vi "ADD to DRIVE.vi"(11 "zero v":T2[](array[typedef])=[{"identifier"=2, "extended?"=FALSE, "type"=0, "payload"=[1, 0, 0, 0, 0, 0, 0]}, {"identifier"=2, "extended?"=FALSE, "type"=0, "payload"=[1]}] {"type" items=["CAN Data", "CAN Remote"]; "identifier" format="%.0x"}) -> (3 "Message Cluster":T1)   [LabVIEW 2015]
uses:
  <vilib>/RioEmbeddedCAN/RioEmbeddedCAN.llb/CANFrameControl.ctl
  PC/QMH Fundamentals - Message Cluster.ctl
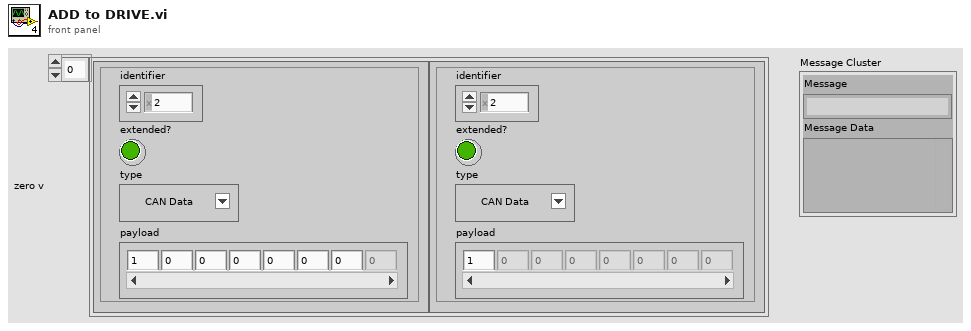
[diagram p1: front panel]
types:
  T1 = typedef "QMH Fundamentals - Message Cluster.ctl" = cluster{"Message":string, "Message Data":variant}
  T2 = typedef "CANFrameControl.ctl" = cluster{"identifier":u32, "extended?":bool, "type":u8, "payload":u8[]}
  T3 = cluster{"Data":cluster{"date/time string":string, "array of cans":cluster{"identifier":u32, "extended?":bool, "type":u8, "payload":u8[]}[]}, "bool":bool}
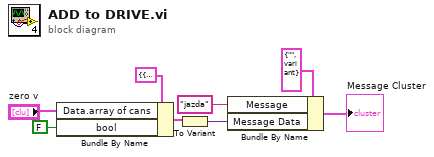
[diagram p0: block diagram]
diagram:
  n1 = Bundle By Name(cluster=T3 {"Data"={"date/time string"="", "array of cans"=[]}, "bool"=TRUE} ("jazda"), "Data.array of cans"="zero v", "bool"=FALSE) -> (w2:T3)
  n2 = To Variant(anything=w2) -> (Variant=w6:variant)
  n3 = Bundle By Name(cluster=T1 {"Message"="", "Message Data"=variant} ("Message Cluster"), "Message"="jazda", "Message Data"=w6) -> (→"Message Cluster":T1)
